vi "Decide Action.vi"(8 "error in (no error)":errorcluster, 11 "Demo Mouse in":refnum<class "Demo Mouse.lvclass">) -> (0 "error out":errorcluster, 2 "Action":T1, 3 "Demo Mouse out":refnum<class "Demo Mouse.lvclass">)   [LabVIEW 2020, in "Demo.lvlib" / "Demo Mouse.lvclass"]
uses:
  Demo Mouse.lvclass
  build/ppl/maze.lvlibp/Action.ctl
  Demo Mouse.lvclass/Demo Mouse.ctl
  build/ppl/maze.lvlibp/Mouse/Mouse.lvclass
  build/ppl/maze.lvlibp
  C:/dev/LabVIEW/Challenges/Maze/build/ppl/maze.lvlibp/Mouse/Mouse.lvclass
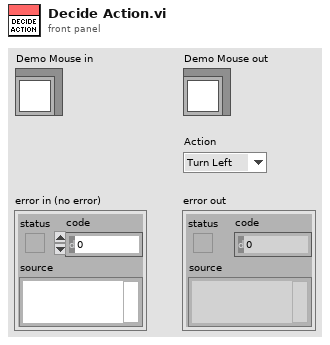
[diagram p1: front panel]
types:
  T1 = typedef "maze.lvlibp/Action.ctl" = enum16{"Turn Left", "Turn Right", "Forward", "*Drop Marker", "*Pickup Marker"}
  T2 = typedef "maze.lvlibp/Distances.ctl" = cluster{"Forward":i32, "Back":i32, "Left":i32, "Right":i32}
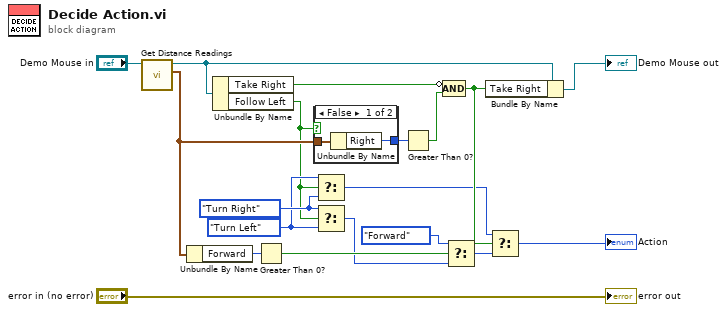
[diagram p0: block diagram]
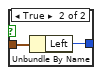
[diagram p2: hidden frame]
diagram:
  w4 = Action."Turn Right" ("Action")
  w3 = Action."Turn Left" ("Action")
  n1 = call "Get Distance Readings.vi"("Mouse in"="Demo Mouse in") -> ("Distances"=w8:T2, "Mouse out"=w12:refnum<class "Demo Mouse.lvclass">)  [unwired: 8 in, 1 out]
  n2 = Unbundle By Name(w8) -> ("Forward"=w17:i32)
  n3 = Unbundle By Name(w12) -> ("Take Right"=w11:bool, "Follow Left"=w2:bool)
  n4 = Greater Than 0?(x=w17) -> (x > 0?=w16:bool)
  n5 = case shown="False" w2 {
    tunnel: w8 -> [w21 w23]
    tunnel: [w20 w22] -> w7
    frame False {
      n6 = Unbundle By Name(w21) -> ("Right"=w20:i32)
    }
    frame True {
      n7 = Unbundle By Name(w23) -> ("Left"=w22:i32)
    }
  }
  n8 = Select(t=w3, s=w2, f=w4) -> (s? t:f=w1:T1)
  n9 = Select(t=w4, s=w2, f=w3) -> (s? t:f=w5:T1)
  n10 = Greater Than 0?(x=w7) -> (x > 0?=w6:bool)
  n11 = Compound Arithmetic op=AND(invert w11, w6) -> (w9:bool)
  n12 = Select(t=Action."Forward" ("Action"), s=w16, f=w5) -> (s? t:f=w14:T1)
  n13 = Bundle By Name(cluster=w12, "Take Right"=w9) -> (→"Demo Mouse out":refnum<class "Demo Mouse.lvclass">)
  n14 = Select(t=w1, s=w9, f=w14) -> (s? t:f=→"Action":T1)
  "error out" <- "error in (no error)"
